vi "MEMR-Find Threshold.vi"(5 "Metrics":dbl[](array[numeric]), 7 "Noise":dbl[](array[numeric]), 9 "Level":dbl[](array[numeric]), 11 "Criterion":dbl) -> (8 "Threshold":dbl)   [LabVIEW 2020]
uses:
  Utility VIs/Math VIs/interp1.vi
  <vilib>/Analysis/NI_AALBase.lvlib
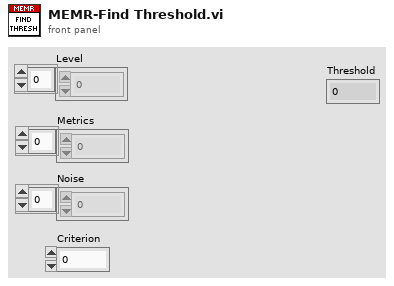
[diagram p1: front panel]
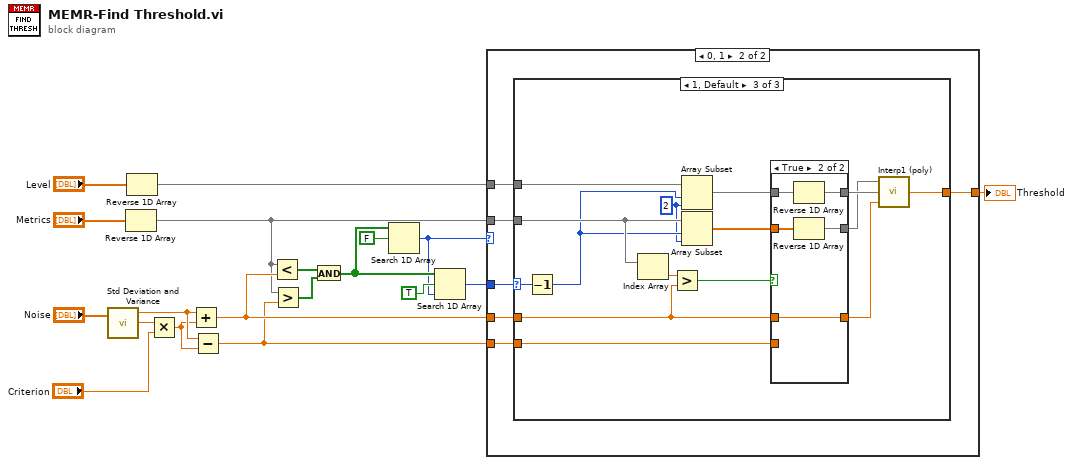
[diagram p0: block diagram]
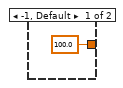
[diagram p2: hidden frame]
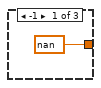
[diagram p3: hidden frame]
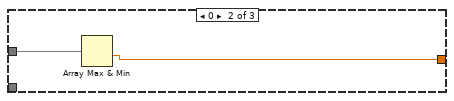
[diagram p4: hidden frame]
diagram:
  n1 = call <vilib>:"Std Deviation and Variance.vi"("X"="Noise") -> ("mean"=w4:dbl, "standard deviation"=w15:dbl)  [unwired: 1 in, 1 out]
  n2 = Reverse 1D Array(array="Metrics") -> (reversed array=w7:dbl[])
  n3 = Reverse 1D Array(array="Level") -> (reversed array=w10:dbl[])
  n4 = Multiply(x=w15, y="Criterion") -> (x*y=w3:dbl)
  n5 = Add(x=w4, y=w3) -> (x+y=w9:dbl)
  n6 = Subtract(x=w4, y=w3) -> (x-y=w8:dbl)
  n7 = Less?(x=w7, y=w9) -> (x < y?=w14:bool[])
  n8 = Greater?(x=w7, y=w8) -> (0:w13:bool[])
  n9 = And(x=w14, y=w13) -> (x .and. y?=w6:bool[])
  n10 = Search 1D Array(1D array=w6, element=FALSE) -> (index of element=w2:i32)  [unwired: 1 in]
  n11 = Search 1D Array(1D array=w6, element=TRUE, start index (0)=w2) -> (index of element=w11:i32)
  n12 = case shown="0, 1" w2 {
    tunnel: [100.0 ("V") w26] -> w16
    tunnel: w11 -> [_ w25]
    tunnel: w10 -> [_ w24]
    tunnel: w9 -> [_ w23]
    tunnel: w8 -> [_ w22]
    tunnel: w7 -> [_ w21]
    frame -1, Default {
    }
    frame 0, 1 {
      n13 = case shown="1, Default" w25 {
        selector: w25 -> [_ _ w43]
        tunnel: [nan w28 w39] -> w26
        tunnel: w24 -> [_ w29 w44]
        tunnel: w21 -> [_ _ w42]
        tunnel: w23 -> [_ _ w40]
        tunnel: w22 -> [_ _ w41]
        frame -1 {
        }
        frame 0 {
          n14 = Array Max & Min(array=w29) -> (min value=w28:dbl)  [unwired: 3 out]
        }
        frame 1, Default {
          w37 = 2 ("length")
          n15 = Decrement(x=w43) -> (x-1=w38:i32)
          n16 = Index Array(array=w42) -> (element=w36:dbl)  [unwired: 1 in]
          n17 = Greater?(x=w36, y=w40) -> (0:w32:bool)
          n18 = Array Subset(array=w44, index=w38, length=w37) -> (w35:dbl[])
          n19 = Array Subset(array=w42, index=w38, length=w37) -> (w34:dbl[])
          n20 = case shown="True" w32 {
            tunnel: w35 -> [w46 w51]
            tunnel: w34 -> [w45 w50]
            tunnel: w41 -> [w47 _]
            tunnel: w40 -> [_ w52]
            tunnel: [w47 w52] -> w33
            tunnel: [w46 w49] -> w31
            tunnel: [w45 w48] -> w30
            frame False {
            }
            frame True {
              n21 = Reverse 1D Array(array=w51) -> (reversed array=w49:dbl[])
              n22 = Reverse 1D Array(array=w50) -> (reversed array=w48:dbl[])
            }
          }
          n23 = call-poly "Interp1 (poly).vi"("X"=w30, "Y"=w31, "U"=w33) -> ("V"=w39:dbl)  [unwired: 2 in]
        }
      }
    }
  }
  "Threshold" <- w16
